vi "LWXPS_GatheringListGet.vi"(0 "XPS Reference IN":refnum<k24>, 11 "LabVIEW error IN":errorcluster) -> (4 "XPS Reference OUT":refnum<k24>, 6 "Returned error code":i32, 8 "Gathering type":string[](array[string]), 10 "XPS Error String":string, 15 "LabVIEW error OUT":errorcluster)   [LabVIEW 2014]
uses:
  D:/XPSQ8_LabView_Library/Development/Source/Dll/Newport.XPS.CommandInterface.dll
  Dll/Newport.XPS.CommandInterface.dll
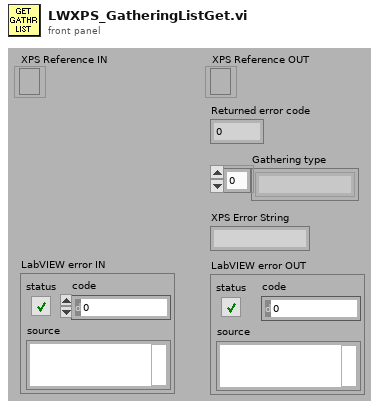
[diagram p1: front panel]
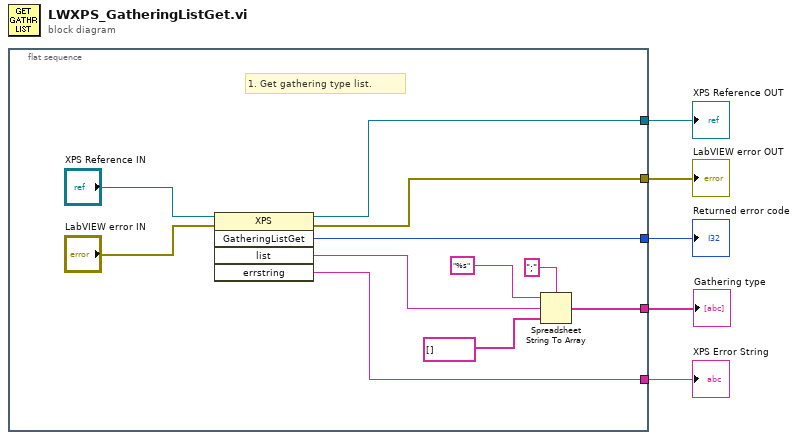
[diagram p0: block diagram]
diagram:
  n1 = flat-sequence {
    tunnel: [w15] -> w5
    tunnel: [w14] -> w4
    tunnel: [w13] -> w3
    tunnel: [w11] -> w2
    tunnel: [w6] -> w1
    frame #0 {
      # "1. Get gathering type list."
      n2 = invoke class="XPS" method="GatheringListGet"(reference="XPS Reference IN", error in="LabVIEW error IN") -> (reference out=w15:refnum<k24>, error out=w14:errorcluster, "GatheringListGet"=w13:i32, "list"=w7:string, "errstring"=w11:string)  [unwired: 3 in]
      n3 = Spreadsheet String To Array(delimiter (Tab)=";" ("Delimiter (Tab)"), format string="%s" ("Format string"), spreadsheet string=w7, array type (2D Dbl)=string[] [] ("Type")) -> (array=w6:string[])
    }
  }
  "XPS Reference OUT" <- w5
  "LabVIEW error OUT" <- w4
  "Returned error code" <- w3
  "XPS Error String" <- w2
  "Gathering type" <- w1
